vi "SVL Limit Testing (waveform) (scalar limits).vi"(8 "error in (no error)":errorcluster, 9 "lower limit":dbl=-inf format="%.2f", 10 "upper limit":dbl=inf format="%.2f", 11 "signal in":waveform(dbl)) -> (0 "error out":errorcluster, 1 "output values":waveform(dbl)[](graph), 2 "test results":bool[](array[boolean]), 3 "test passed?":bool)   [LabVIEW 2017, in "SoundVib_LimitTest.lvlib"]
doc: "Performs limit testing on waveforms, spectra, XY data, identified peaks, or scalar measurements. You can specify an upper and lower boundary of the envelope to define a pass range. This VI uses the defined pass range to test the input signal. VI outputs apply only to the current input signal. You can wire output values to a graph to view the limits, signal, and failures. Wire data to the<B> signal in</B> input to determine the polymorphic instance to use or manually select the instance."
uses:
  <vilib>/addons/Sound and Vibration/svt_Limit Test/SoundVib_LimitTest.lvlib
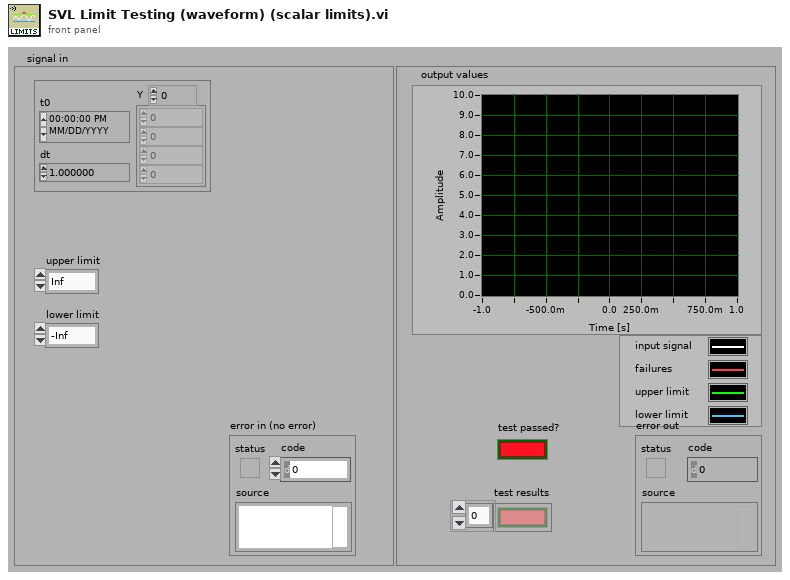
[diagram p1: front panel]
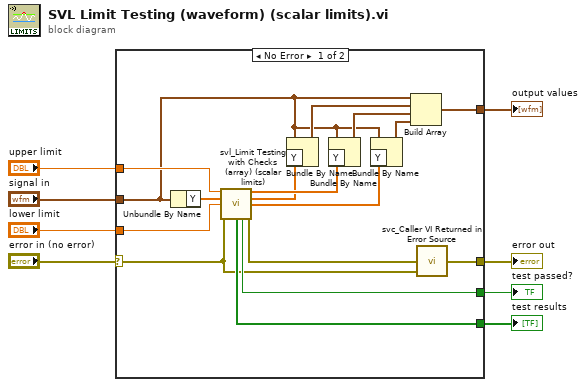
[diagram p0: block diagram]
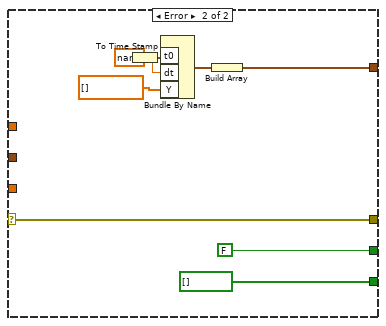
[diagram p2: hidden frame]
diagram:
  n1 = case shown="No Error" "error in (no error)" {
    selector: "error in (no error)" -> [w9 w32]
    tunnel: [w24 w32] -> w7
    tunnel: "upper limit" -> [w21 _]
    tunnel: "signal in" -> [w16 _]
    tunnel: "lower limit" -> [w22 _]
    tunnel: [w17 w26] -> w3
    tunnel: [w11 bool[] [] ("Array Constant")] -> w2
    tunnel: [w10 FALSE] -> w1
    frame No Error {
      n2 = Unbundle By Name(w16) -> ("Y"=w23:dbl[])
      n3 = call <vilib>:"svl_Limit Testing with Checks (array) (scalar limits).vi"("upper limit"=w21, "input array"=w23, "lower limit"=w22, "error in (no error)"=w9) -> ("upper limit array"=w15:dbl[], "failure array"=w14:dbl[], "lower limit array"=w13:dbl[], "test results"=w11:bool[], "test passed"=w10:bool, "error out"=w12:errorcluster)  [unwired: 6 in]
      n4 = Bundle By Name(cluster=w16, "Y"=w14) -> (w20:waveform(dbl))
      n5 = Bundle By Name(cluster=w16, "Y"=w15) -> (w19:waveform(dbl))
      n6 = Bundle By Name(cluster=w16, "Y"=w13) -> (w18:waveform(dbl))
      n7 = Build Array(w16, w20, w19, w18) -> (w17:waveform(dbl)[])
      n8 = call <vilib>:"svc_Caller VI Returned in Error Source.vi"("warning input to caller"=w9, "error in (no error)"=w12) -> ("error out"=w24:errorcluster)  [unwired: 3 in]
    }
    frame Error {
      w29 = nan ("t0")
      n9 = To Time Stamp(1:w29) -> (0:w25:timestamp)
      n10 = Bundle By Name("t0"=w25, "dt"=w29, "Y"=dbl[] []) -> (w27:waveform(dbl))  [unwired: 1 in]
      n11 = Build Array(w27) -> (w26:waveform(dbl)[])
    }
  }
  "error out" <- w7
  "output values" <- w3
  "test passed?" <- w1
  "test results" <- w2
